vi "BT 打印全流程.vi"(0 "文件路径":path, 1 "BT 具名数据源名称":string[](array[string]), 2 "输入内容":string[](array[string]), 3 "error in (no error)":errorcluster caption="错误输入（无错误）") -> (10 "error out":errorcluster caption="错误输出")   [LabVIEW 2023]
panel:
  in  "BarTender.IBtApplication":refnum<k7>
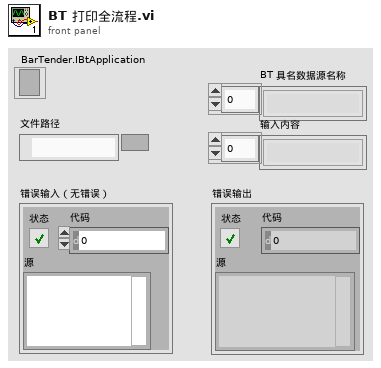
[diagram p1: front panel]
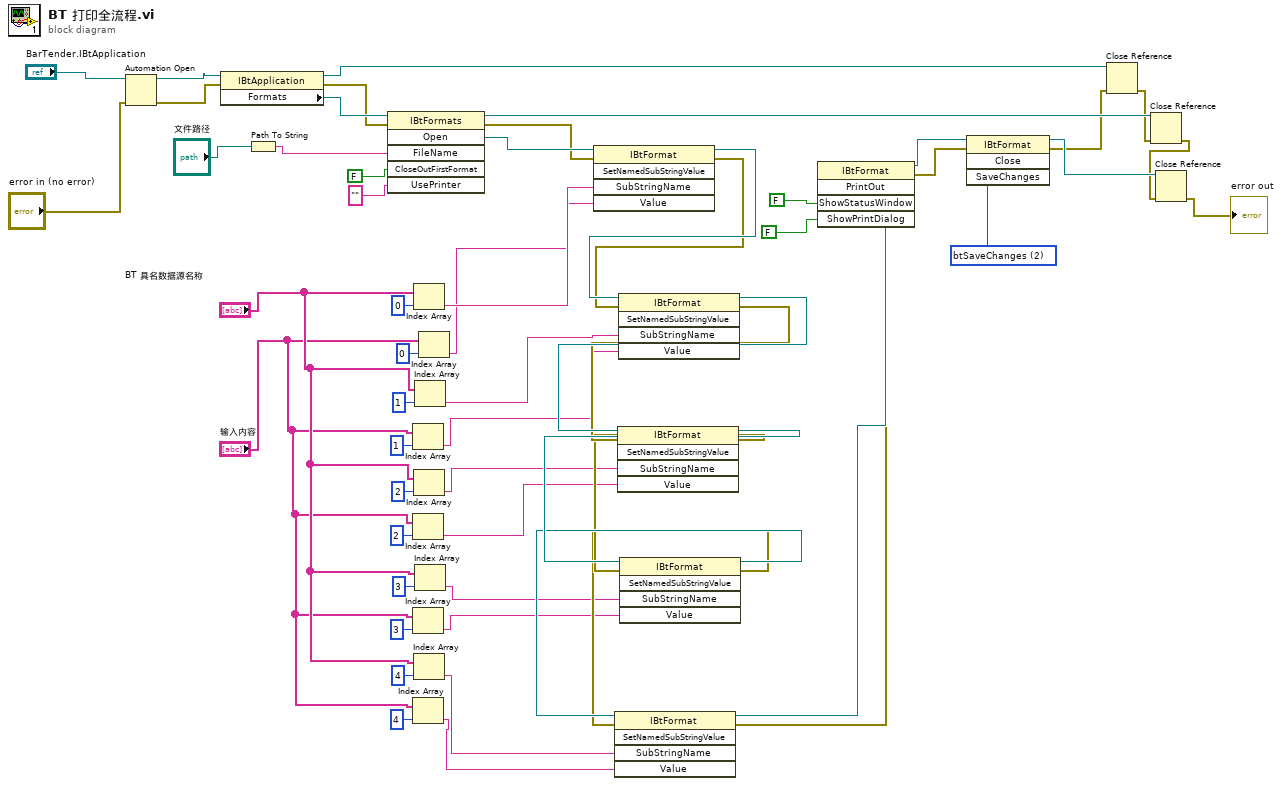
[diagram p0: block diagram]
diagram:
  w43 = 2 items=["btPromptSave", "btDoNotSaveChanges", "btSaveChanges"] ("SaveChanges")
  n1 = Automation Open(error in (no error)="error in (no error)", Automation Refnum="BarTender.IBtApplication") -> (Automation Refnum=w55:refnum<k7>, error out=w54:errorcluster)  [unwired: 2 in]
  n2 = property class="IBtApplication"(reference=w55, error in=w54) -> (reference out=w49:refnum<k7>, error out=w50:errorcluster, "Formats"=w53:refnum<k7>)
  n3 = Path To String(path="文件路径") -> (string=w45:string)
  n4 = invoke class="IBtFormats" method="Open"(reference=w53, error in=w50, "FileName"=w45, "CloseOutFirstFormat"=FALSE, "UsePrinter"="") -> (reference out=w48:refnum<k7>, error out=w33:errorcluster, "Open"=w34:refnum<k7>)  [unwired: 1 in, 3 out]
  n5 = Index Array(array="输入内容", index=1) -> (element=w7:string)
  n6 = Index Array(array="输入内容", index=2) -> (element=w5:string)
  n7 = Index Array(array="输入内容", index=3) -> (element=w3:string)
  n8 = Index Array(array="输入内容", index=4) -> (element=w1:string)
  n9 = Index Array(array="BT 具名数据源名称", index=0) -> (element=w21:string)
  n10 = Index Array(array="BT 具名数据源名称", index=2) -> (element=w6:string)
  n11 = Index Array(array="BT 具名数据源名称", index=4) -> (element=w2:string)
  n12 = Index Array(array="BT 具名数据源名称", index=1) -> (element=w8:string)
  n13 = Index Array(array="BT 具名数据源名称", index=3) -> (element=w4:string)
  n14 = Index Array(array="输入内容", index=0) -> (element=w20:string)
  n15 = invoke class="IBtFormat" method="SetNamedSubStringValue"(reference=w34, error in=w33, "SubStringName"=w21, "Value"=w20) -> (reference out=w32:refnum<k7>, error out=w27:errorcluster)  [unwired: 1 in, 3 out]
  n16 = invoke class="IBtFormat" method="SetNamedSubStringValue"(reference=w32, error in=w27, "SubStringName"=w8, "Value"=w7) -> (reference out=w31:refnum<k7>, error out=w26:errorcluster)  [unwired: 1 in, 3 out]
  n17 = invoke class="IBtFormat" method="SetNamedSubStringValue"(reference=w31, error in=w26, "SubStringName"=w6, "Value"=w5) -> (reference out=w30:refnum<k7>, error out=w25:errorcluster)  [unwired: 1 in, 3 out]
  n18 = invoke class="IBtFormat" method="SetNamedSubStringValue"(reference=w30, error in=w25, "SubStringName"=w4, "Value"=w3) -> (reference out=w29:refnum<k7>, error out=w24:errorcluster)  [unwired: 1 in, 3 out]
  n19 = invoke class="IBtFormat" method="SetNamedSubStringValue"(reference=w29, error in=w24, "SubStringName"=w2, "Value"=w1) -> (reference out=w28:refnum<k7>, error out=w23:errorcluster)  [unwired: 1 in, 3 out]
  n20 = invoke class="IBtFormat" method="PrintOut"(reference=w28, error in=w23, "ShowStatusWindow"=FALSE, "ShowPrintDialog"=FALSE) -> (reference out=w36:refnum<k7>, error out=w35:errorcluster)  [unwired: 1 in, 3 out]
  n21 = invoke class="IBtFormat" method="Close"(reference=w36, error in=w35, "SaveChanges"=w43) -> (reference out=w42:refnum<k7>, error out=w41:errorcluster)  [unwired: 1 in, 2 out]
  n22 = Close Reference(reference=w49, error in (no error)=w41) -> (error out=w47:errorcluster)
  n23 = Close Reference(reference=w48, error in (no error)=w47) -> (error out=w40:errorcluster)
  n24 = Close Reference(reference=w42, error in (no error)=w40) -> (error out=→"error out":errorcluster)
